vi "BN_outputLayer.vi"(0 "Target_outX":dbl[](array[numeric]), 1 "Out_hx":dbl[](array[numeric]), 2 "Out_outX":dbl[](array[numeric]), 3 "Learning rate":dbl, 4 "Weights_outX_IN":dbl[][](array[numeric])) -> (5 "Weights_outX_OUT":dbl[][](array[numeric]))   [LabVIEW 2016]
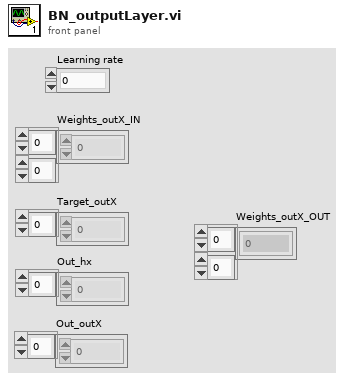
[diagram p1: front panel]
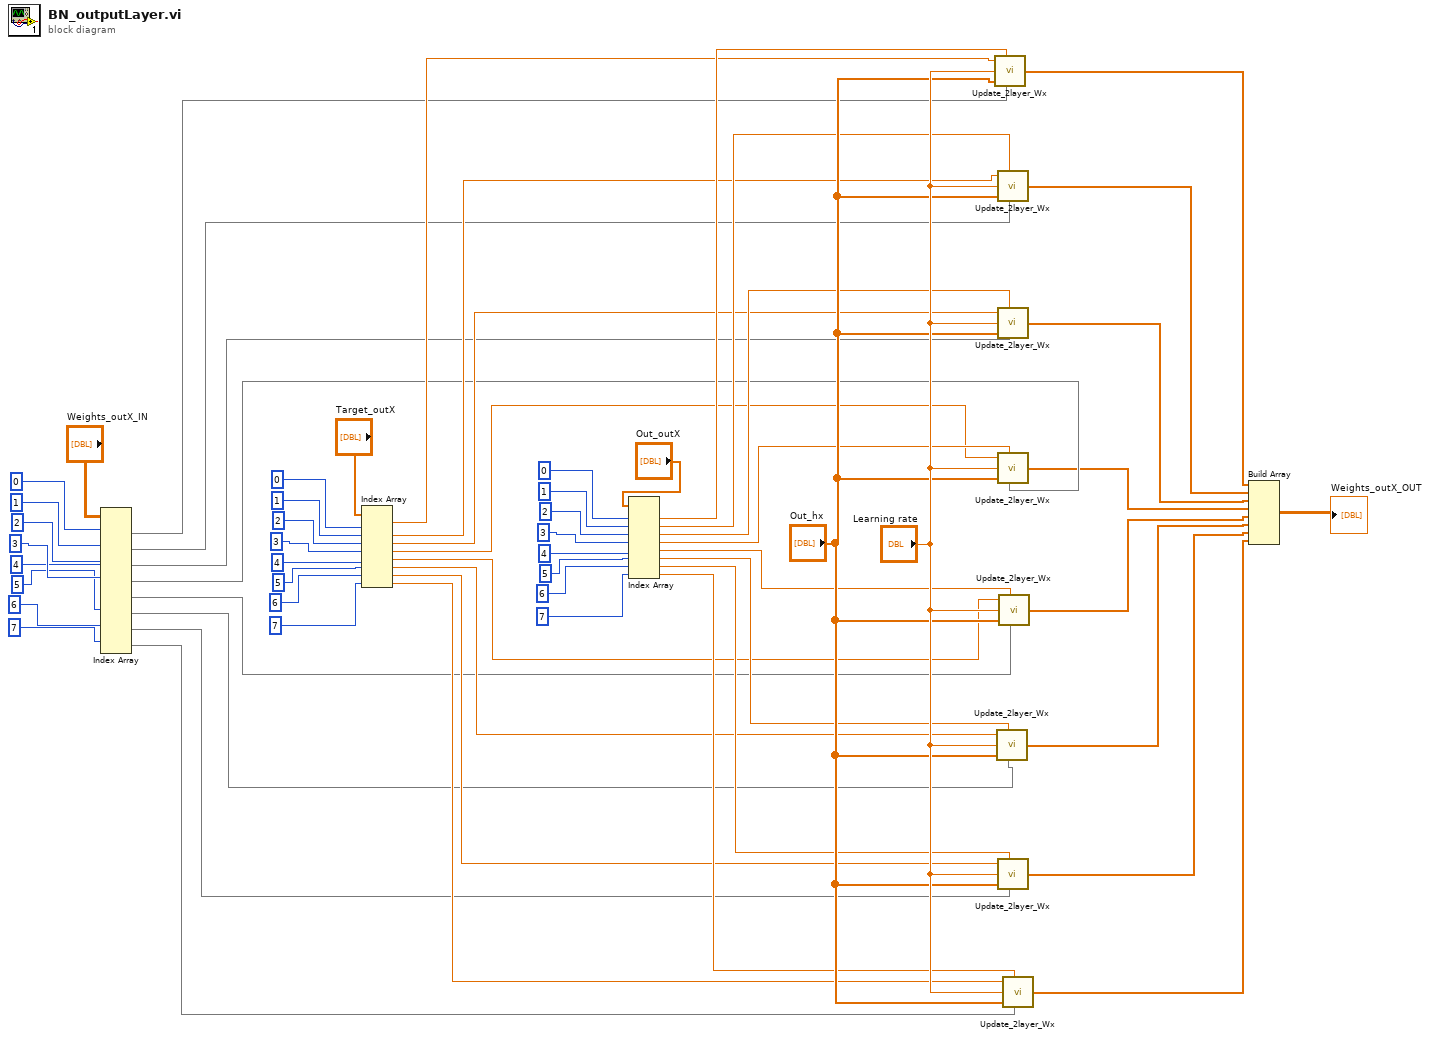
[diagram p0: block diagram]
diagram:
  n1 = Index Array(array="Weights_outX_IN", index (row) #1=0 ("index"), index (row) #2=1 ("index"), index (row) #3=2 ("index"), index (row) #4=3 ("index"), index (row) #5=4 ("index"), index (row) #6=5 ("index"), index (row) #7=6 ("index"), index (row) #8=7 ("index")) -> (element #1=w17:dbl[], element #2=w16:dbl[], element #3=w15:dbl[], element #4=w14:dbl[], element #5=w13:dbl[], element #6=w12:dbl[], element #7=w11:dbl[], element #8=w10:dbl[])  [unwired: 8 in]
  n2 = Index Array(array="Target_outX", index #1=0 ("index"), index #2=1 ("index"), index #3=2 ("index"), index #4=3 ("index"), index #5=4 ("index"), index #6=5 ("index"), index #7=6 ("index"), index #8=7 ("index")) -> (element #1=w34:dbl, element #2=w33:dbl, element #3=w32:dbl, element #4=w31:dbl, element #5=w30:dbl, element #6=w29:dbl, element #7=w28:dbl, element #8=w27:dbl)
  n3 = Index Array(array="Out_outX", index #1=0 ("index"), index #2=1 ("index"), index #3=2 ("index"), index #4=3 ("index"), index #5=4 ("index"), index #6=5 ("index"), index #7=6 ("index"), index #8=7 ("index")) -> (element #1=w51:dbl, element #2=w50:dbl, element #3=w49:dbl, element #4=w48:dbl, element #5=w47:dbl, element #6=w46:dbl, element #7=w45:dbl, element #8=w44:dbl)
  n4 = call "Update_2layer_Wx.vi"("Target_OutX"=w34, "2layer_OutX 2"=w51, "Learning rate"="Learning rate", "Array_Out_hx"="Out_hx", "Weights_2layer"=w17) -> ("Weights_2layer_updated"=w9:dbl[])
  n5 = call "Update_2layer_Wx.vi"("Target_OutX"=w29, "2layer_OutX 2"=w46, "Learning rate"="Learning rate", "Array_Out_hx"="Out_hx", "Weights_2layer"=w12) -> ("Weights_2layer_updated"=w4:dbl[])
  n6 = call "Update_2layer_Wx.vi"("Target_OutX"=w33, "2layer_OutX 2"=w50, "Learning rate"="Learning rate", "Array_Out_hx"="Out_hx", "Weights_2layer"=w16) -> ("Weights_2layer_updated"=w8:dbl[])
  n7 = call "Update_2layer_Wx.vi"("Target_OutX"=w32, "2layer_OutX 2"=w49, "Learning rate"="Learning rate", "Array_Out_hx"="Out_hx", "Weights_2layer"=w15) -> ("Weights_2layer_updated"=w7:dbl[])
  n8 = call "Update_2layer_Wx.vi"("Target_OutX"=w31, "2layer_OutX 2"=w48, "Learning rate"="Learning rate", "Array_Out_hx"="Out_hx", "Weights_2layer"=w14) -> ("Weights_2layer_updated"=w6:dbl[])
  n9 = call "Update_2layer_Wx.vi"("Target_OutX"=w28, "2layer_OutX 2"=w45, "Learning rate"="Learning rate", "Array_Out_hx"="Out_hx", "Weights_2layer"=w11) -> ("Weights_2layer_updated"=w3:dbl[])
  n10 = call "Update_2layer_Wx.vi"("Target_OutX"=w30, "2layer_OutX 2"=w47, "Learning rate"="Learning rate", "Array_Out_hx"="Out_hx", "Weights_2layer"=w13) -> ("Weights_2layer_updated"=w5:dbl[])
  n11 = call "Update_2layer_Wx.vi"("Target_OutX"=w27, "2layer_OutX 2"=w44, "Learning rate"="Learning rate", "Array_Out_hx"="Out_hx", "Weights_2layer"=w10) -> ("Weights_2layer_updated"=w2:dbl[])
  n12 = Build Array(w9, w8, w7, w6, w5, w4, w3, w2) -> (→"Weights_outX_OUT":dbl[][])
